vi "Write Trace Level.vi"(8 "error in (no error)":errorcluster, 10 "Trace Level":T1, 11 "Command Processor Actor in":refnum<class "Command Processor Actor.lvclass">) -> (0 "error out":errorcluster, 3 "Command Processor Actor out":refnum<class "Command Processor Actor.lvclass">)   [LabVIEW 2014, in "Robot Actor Framework.lvlib" / "Command Processor Actor.lvlib" / "Command Processor Actor.lvclass"]
uses:
  Command Processor Actor.lvclass
  Trace/Trace Class/Trace Levels.ctl
  Command Processor Actor.lvclass/Command Processor Actor.ctl
  Trace/Trace Class/Trace.lvclass
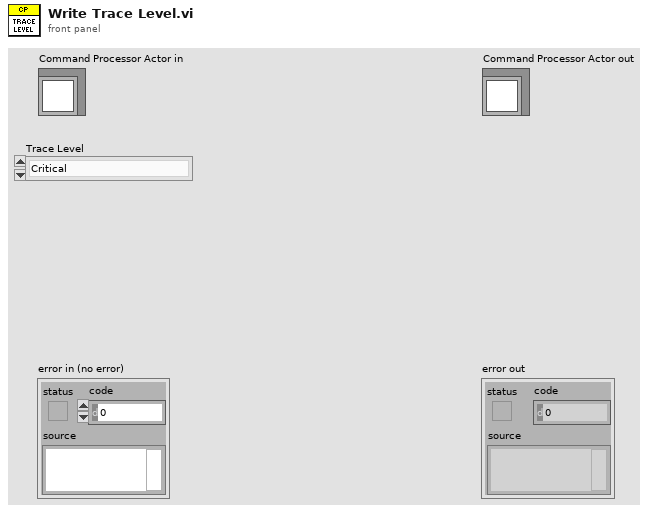
[diagram p1: front panel]
types:
  T1 = typedef "Robot Actor Framework.lvlib/Trace.lvlib/Trace.lvclass/Trace Levels.ctl" = enum16{"Critical", "Error", "Warning", "Informational", "Debug"}
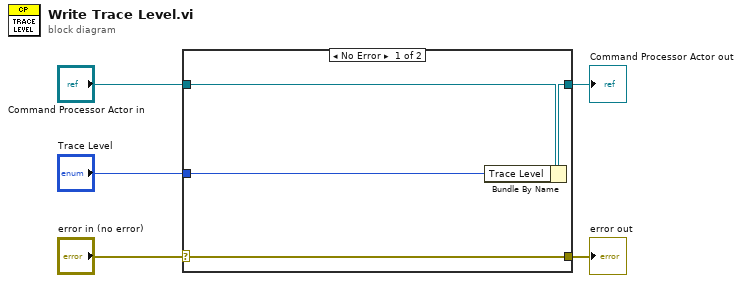
[diagram p0: block diagram]
diagram:
  n1 = case shown="No Error" "error in (no error)" {
    selector: "error in (no error)" -> [w9 w10]
    tunnel: [w9 w10] -> w4
    tunnel: [w7 w11] -> w2
    tunnel: "Command Processor Actor in" -> [w8 w11]
    tunnel: "Trace Level" -> [w6 _]
    frame No Error {
      n2 = Bundle By Name(cluster=w8, "Trace Level"=w6) -> (w7:refnum<class "Command Processor Actor.lvclass">)
    }
    frame Error {
    }
  }
  "error out" <- w4
  "Command Processor Actor out" <- w2
